vi "ACT LG Add to Log File.vi"(0 "Directory Log Path":path, 1 "File Refnum In":refnum<file>, 2 "Header Text":string, 7 "Line To Append":string, 11 "Error in (no error)":errorcluster, 12 "Append Mode (new line)":T1=enum."New Line", 13 "Size Limit (250 KB)":dbl=250.0 format="%.2f", 14 "Timestamp (t:yes)":bool=TRUE) -> (3 "File Refnum Out":refnum<file>, 4 "Logged Line":string, 6 "Current File Size":dbl=250.0 format="%.2f", 15 "Error out":errorcluster)   [LabVIEW 2012]
doc: "This VI is used for the purpose of logging data to a file. The \"Directory Log Name\" should contain the directory name that you want your log files to be placed. This directory MUST have a \"_\" (i.e., \"underscore\") contained in it. An example would be: BEESON_DIR. The VI checks to see if your directory is valid and then will name all of your logfiles \"BEESON_[n].log\" were \"n\" is a U32 integer pertaining to the order in which the file was created. A new logfile will dynamically be created based on the current logfile's size in comparison to the \"Size Limit.\" The most recent logfile will always be filled to capacity before the next one is created.\n\nIf files are deleted from the logfile directory in use then the vi will create a file next in the sequence of previously used numbers.\n\nThis scheme of logging data will support 4,294,967,295 files per directory, and at 250k a piece will top out at around 1,000 Tera-Bytes Maximum--well beyond any PCs capabilities! So delete old files before your disk becomes full.\n\nThis vi was created by David Gianetto, contact me with any problems, questions, etc."
uses:
  File IO/Type Defs/FILE New Line Enum.ctl
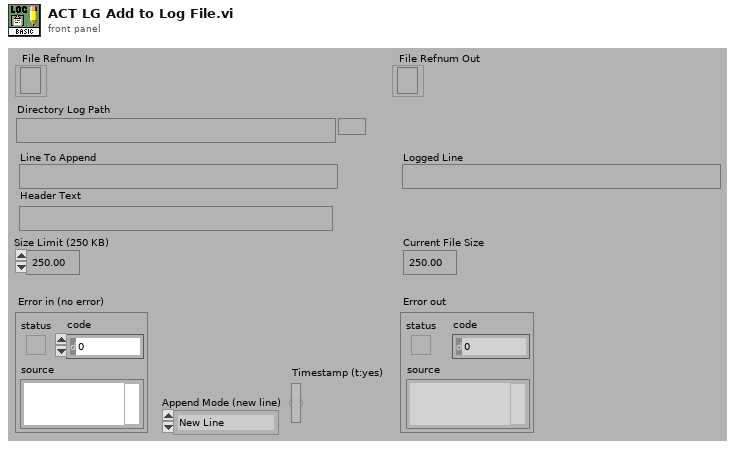
[diagram p1: front panel]
types:
  T1 = typedef "FILE New Line Enum.ctl" = enum16{"No New Line", "New Line"}
  T2 = enum16{"open", "replace", "create", "open or create", "replace or create", "replace or create with confirmation"}
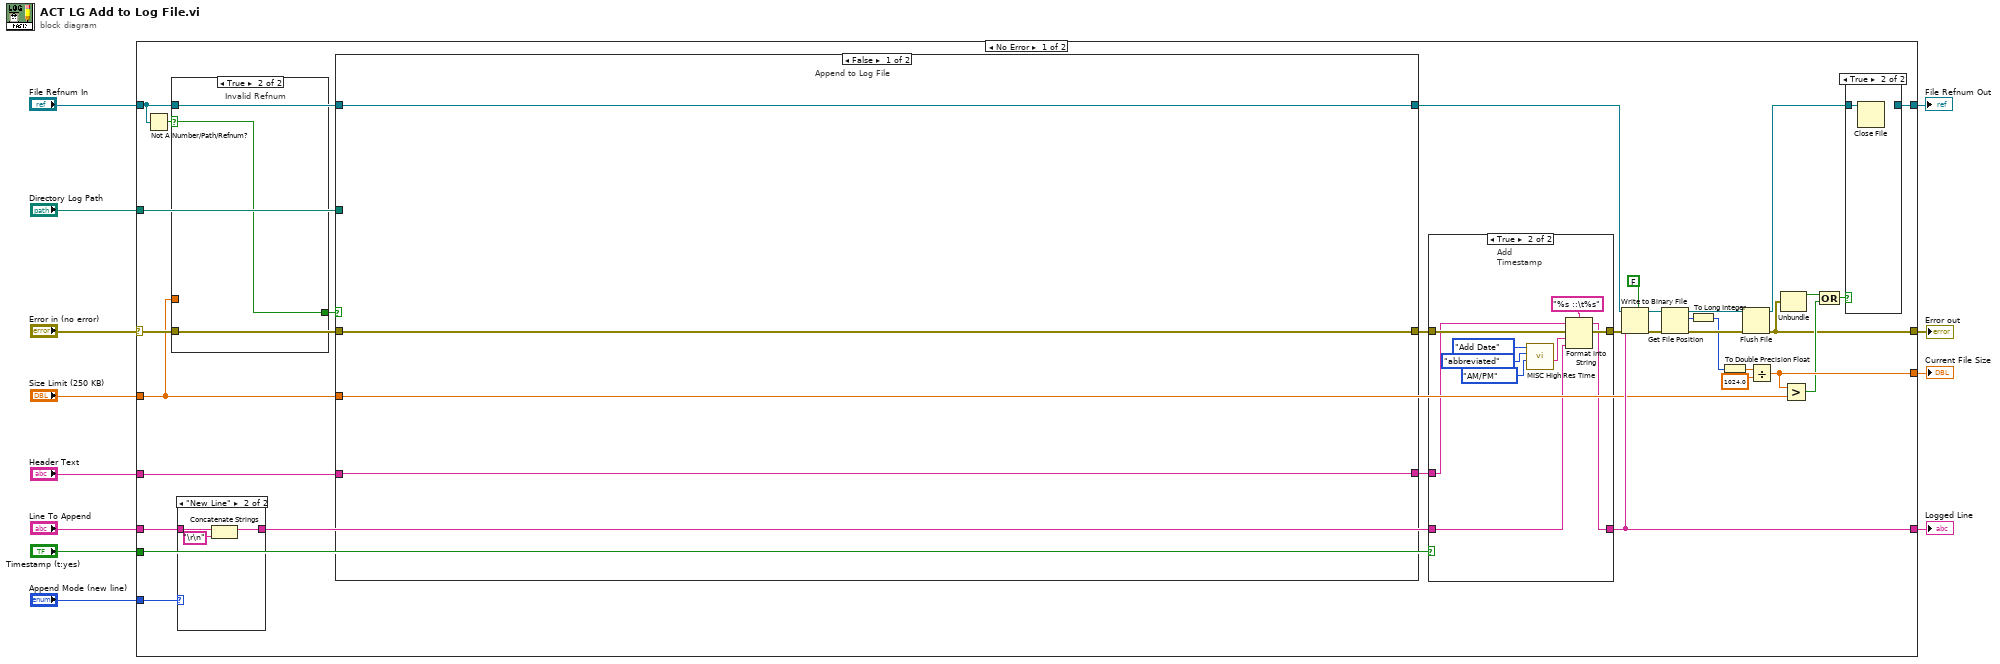
[diagram p0: block diagram]
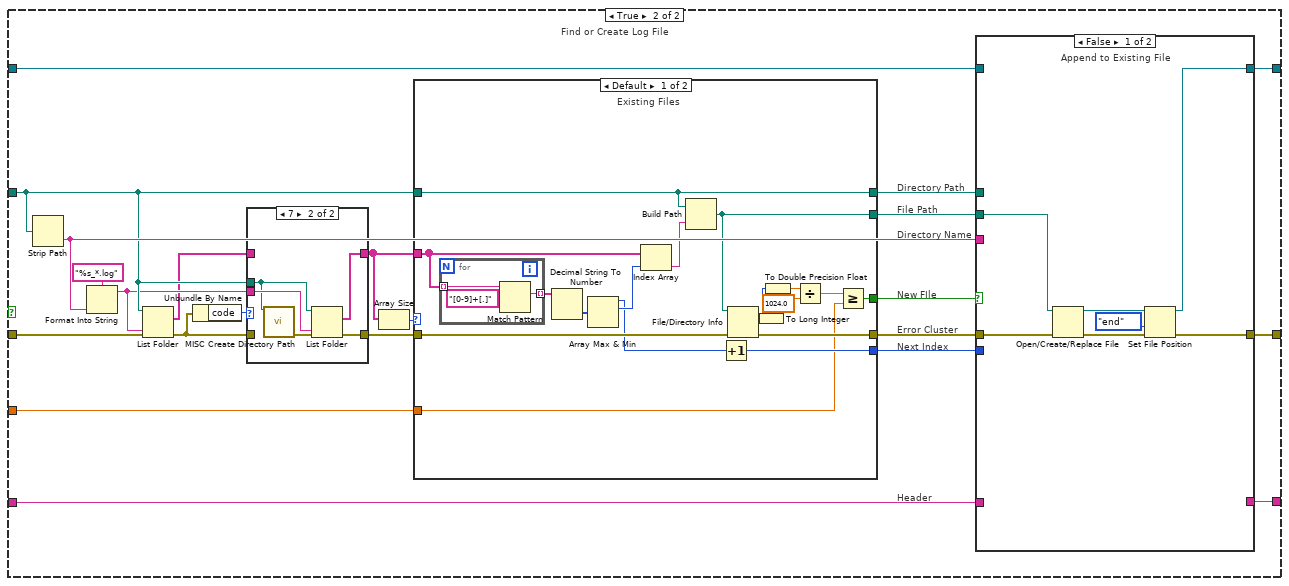
[diagram p3: hidden frame]
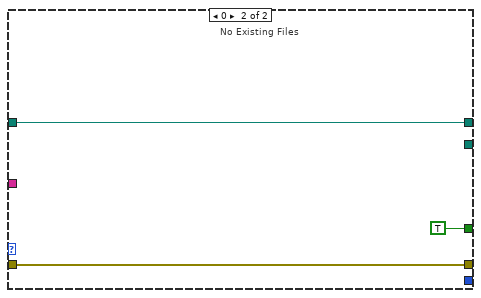
[diagram p5: hidden frame]
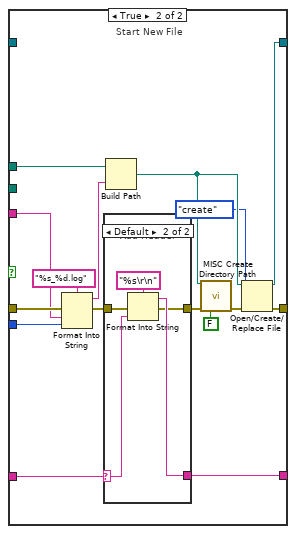
[diagram p6: hidden frame]
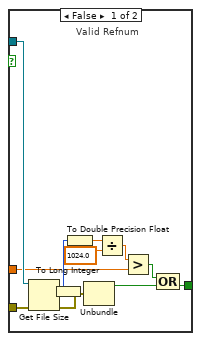
[diagram p8: hidden frame]
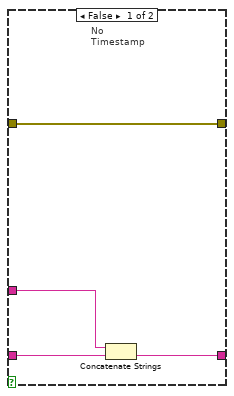
[diagram p10: hidden frame]
diagram:
  n1 = case shown="No Error" "Error in (no error)" {
    selector: "Error in (no error)" -> [w30 w164]
    tunnel: "Line To Append" -> [w23 _]
    tunnel: "Directory Log Path" -> [w41 _]
    tunnel: "Size Limit (250 KB)" -> [w26 _]
    tunnel: [w20 w164] -> w11
    tunnel: [w27 _] -> w10
    tunnel: "Header Text" -> [w43 _]
    tunnel: [w37 _] -> w8
    tunnel: "Timestamp (t:yes)" -> [w42 _]
    tunnel: "Append Mode (new line)" -> [w21 _]
    tunnel: [w35 w163] -> w2
    tunnel: "File Refnum In" -> [w29 w163]
    frame No Error {
      n2 = Not A Number/Path/Refnum?(number/path/refnum=w29) -> (NaN/Path/Refnum?=w31:bool)
      n3 = case shown="True" w31 {
        selector: w31 -> [_ w146]
        tunnel: w30 -> [w145 _]
        tunnel: [w135 w146] -> w28
        tunnel: w29 -> [w140 _]
        tunnel: w26 -> [w138 _]
        frame False {
          # "Valid Refnum"
          n4 = Get File Size(file=w140, error in=w145) -> (size (in bytes)=w134:i64, 0:w144:errorcluster)  [unwired: 1 out]
          n5 = To Long Integer(number=w134) -> (32bit integer=w141:i32)
          n6 = To Double Precision Float(number=w141) -> (double precision float=w142:dbl)
          n7 = Unbundle(w144) -> ("status"=w136:bool)  [unwired: 2 out]
          n8 = Divide(x=w142, y=1024.0) -> (x/y=w139:dbl)
          n9 = Greater?(x=w139, y=w138) -> (0:w137:bool)
          n10 = Compound Arithmetic op=OR(w137, w136) -> (w135:bool)
        }
        frame True {
          # "Invalid Refnum"
        }
      }
      n11 = case shown="\"New Line\"" w21 {
        tunnel: w23 -> [w45 w48]
        tunnel: [w45 w47] -> w22
        frame "No New Line" {
        }
        frame "New Line" {
          n12 = Concatenate Strings(w48, "\r\n") -> (w47:string)
        }
      }
      n13 = case shown="False" w28 {
        tunnel: [w50 w70] -> w44
        tunnel: w43 -> [w51 w69]
        tunnel: w41 -> [_ w65]
        tunnel: [w51 w64] -> w36
        tunnel: w26 -> [_ w63]
        tunnel: w30 -> [w50 w62]
        tunnel: w29 -> [w49 w61]
        tunnel: [w49 w52] -> w17
        frame False {
          # "Append to Log File"
        }
        frame True {
          # "Find or Create Log File"
          # "Header"
          # "Next Index"
          # "Error Cluster"
          # "New FIle"
          # "Directory Name"
          # "File Path"
          # "Directory Path"
          n14 = Strip Path(path=w65) -> (name=w68:string)  [unwired: 1 out]
          n15 = Format Into String(format string="%s_*.log", w68) -> (resulting string=w55:string)  [unwired: 2 in, 1 out]
          n16 = List Folder(path=w65, pattern=w55, error in=w62) -> (filenames=w54:string[], error out=w56:errorcluster)  [unwired: 3 out]
          n17 = Unbundle By Name(w56) -> ("code"=w57:i32)
          n18 = case shown="7" w57 {
            tunnel: [w75 w79] -> w58
            tunnel: w56 -> [w75 _]
            tunnel: w65 -> [_ w76]
            tunnel: w55 -> [_ w78]
            tunnel: [w74 w77] -> w53
            tunnel: w54 -> [w74 _]
            frame Default {
            }
            frame 7 {
              n19 = call "MISC Create Directory Path.vi"("Path"=w76) -> ("Error Out"=w80:errorcluster)  [unwired: 2 in, 12 out]
              n20 = List Folder(path=w76, pattern=w78, error in=w80) -> (filenames=w77:string[], error out=w79:errorcluster)  [unwired: 3 out]
            }
          }
          n21 = Array Size(array=w53) -> (size(s)=w59:i32)
          n22 = case shown="Default" w59 {
            tunnel: w53 -> [w91 _]
            tunnel: [w98 w104] -> w71
            tunnel: w65 -> [w85 w103]
            tunnel: [w86 _] -> w72
            tunnel: [w90 _] -> w73
            tunnel: w58 -> [w97 w104]
            tunnel: [w85 w103] -> w67
            tunnel: w63 -> [w83 _]
            tunnel: [w82 TRUE] -> w66
            frame Default {
              # "Existing Files"
              n23 = for {
                tunnel: w91 -> [w101] mode=indexing
                tunnel: [w99] -> w89 mode=indexing
                n24 = Match Pattern(string=w101, regular expression="[0-9]+[.]") -> (match substring=w99:string)  [unwired: 4 out]
              }
              n25 = Decimal String To Number(string=w89) -> (number=w88:i32[])  [unwired: 3 out]
              n26 = Array Max & Min(array=w88) -> (max value=w87:i32, max index (indices)=w95:i32)  [unwired: 2 out]
              n27 = Index Array(array=w91, index=w95) -> (element=w96:string)
              n28 = Build Path(base path=w85, name or relative path=w96) -> (appended path=w90:path)
              n29 = Increment(x=w87) -> (x+1=w86:i32)
              n30 = File/Directory Info(path=w90, error in=w97) -> (size=w81:i64, error out=w98:errorcluster)  [unwired: 5 out]
              n31 = To Long Integer(number=w81) -> (32bit integer=w94:i32)
              n32 = To Double Precision Float(number=w94) -> (double precision float=w93:dbl)
              n33 = Divide(x=w93, y=1024.0) -> (x/y=w84:dbl)
              n34 = Greater Or Equal?(x=w84, y=w83) -> (x >= y?=w82:bool)
            }
            frame 0 {
              # "No Existing Files"
            }
          }
          n35 = case shown="False" w66 {
            tunnel: w73 -> [w110 _]
            tunnel: w72 -> [_ w123]
            tunnel: w68 -> [_ w125]
            tunnel: w69 -> [_ w124]
            tunnel: w71 -> [w111 w126]
            tunnel: [w107 w118] -> w70
            tunnel: w67 -> [_ w120]
            tunnel: [_ w119] -> w64
            tunnel: [w105 w117] -> w52
            tunnel: w61 -> [_ _]
            frame False {
              # "Append to Existing File"
              n36 = Open/Create/Replace File(file path (use dialog)=w110, error in=w111) -> (refnum out=w106:refnum<file>, error out=w108:errorcluster)  [unwired: 5 out]
              n37 = Set File Position(refnum=w106, from (0:start)=enum16{"start", "end", "current"}."end" ("pos mode (0:2)"), error in=w108) -> (refnum out=w105:refnum<file>, error out=w107:errorcluster)  [unwired: 1 out]
            }
            frame True {
              # "Start New File"
              n38 = Format Into String(format string="%s_%d.log", error in=w126, w125, w123) -> (resulting string=w121:string, error out=w127:errorcluster)  [unwired: 1 in]
              n39 = case shown="Default" w124 {
                selector: w124 -> [_ w132]
                tunnel: [w128 w129] -> w116
                tunnel: w127 -> [w128 w133]
                tunnel: [_ w130] -> w119
                frame "" {
                  # "No Header"
                }
                frame Default {
                  # "Add Header"
                  n40 = Format Into String(format string="%s\r\n", error in=w133, w132) -> (resulting string=w130:string, error out=w129:errorcluster)  [unwired: 1 in]
                }
              }
              n41 = Build Path(base path=w120, name or relative path=w121) -> (appended path=w114:path)
              n42 = call "MISC Create Directory Path.vi"("Path"=w114, "Error In (no error)"=w116, "Input Type (T:Directories only)"=FALSE) -> ("Error Out"=w115:errorcluster)  [unwired: 12 out]
              n43 = Open/Create/Replace File(file path (use dialog)=w114, error in=w115, operation (0:open)=T2."create") -> (refnum out=w117:refnum<file>, error out=w118:errorcluster)  [unwired: 4 out]
            }
          }
        }
      }
      n44 = case shown="True" w42 {
        tunnel: w22 -> [w150 w162]
        tunnel: w44 -> [w152 w161]
        tunnel: [w152 w160] -> w38
        tunnel: [w149 w159] -> w37
        tunnel: w36 -> [w151 w153]
        frame False {
          # "No\nTimestamp"
          n45 = Concatenate Strings(w151, w150) -> (w149:string)
        }
        frame True {
          # "Add\nTimestamp"
          n46 = call "MISC High Res Time.vi"("Time Standard (am/pm)"=enum16{"AM/PM", "24 Hour"}."AM/PM", "Date Format (Abb)"=enum16{"short", "long", "abbreviated"}."abbreviated" ("date format (abbreviated)"), "Mode (add date)"=enum16{"Add Date", "Time Only"}."Add Date") -> ("Date/Time String"=w154:string)  [unwired: 6 out]
          n47 = Format Into String(format string="%s ::\t%s", initial string=w153, error in=w161, w154, w162) -> (resulting string=w159:string, error out=w160:errorcluster)
        }
      }
      n48 = Write to Binary File(file (use dialog)=w17, data=w37, error in=w38, 5:FALSE ("prepend array or string size? (T)")) -> (refnum out=w16:refnum<file>, error out=w15:errorcluster)  [unwired: 3 out]
      n49 = Get File Position(4:w15, 7:w16) -> (0:w40:errorcluster, 2:w14:i64, 3:w39:refnum<file>)
      n50 = To Long Integer(number=w14) -> (32bit integer=w32:i32)
      n51 = To Double Precision Float(number=w32) -> (double precision float=w33:dbl)
      n52 = Flush File(refnum=w39, error in=w40) -> (refnum out=w18:refnum<file>, error out=w20:errorcluster)
      n53 = Divide(x=w33, y=1024.0) -> (x/y=w27:dbl)
      n54 = Unbundle(w20) -> ("status"=w25:bool)  [unwired: 2 out]
      n55 = Greater?(x=w27, y=w26) -> (0:w24:bool)
      n56 = Compound Arithmetic op=OR(w25, w24) -> (w19:bool)
      n57 = case shown="True" w19 {
        tunnel: [w147 _] -> w35
        tunnel: w18 -> [w147 w148]
        frame False {
        }
        frame True {
          n58 = Close File(refnum=w148) -> ()  [unwired: 1 in, 2 out]
        }
      }
    }
    frame Error {
    }
  }
  "Error out" <- w11
  "Current File Size" <- w10
  "Logged Line" <- w8
  "File Refnum Out" <- w2
